vi "handle HTTP Error.vi"(8 "Status String":string, 9 "status code":u16, 11 "error in (no error)":errorcluster) -> (1 "status code dup":u16, 3 "error out":errorcluster)   [LabVIEW 2025, in "http-client.lvclass"]
uses:
  http-client.lvclass
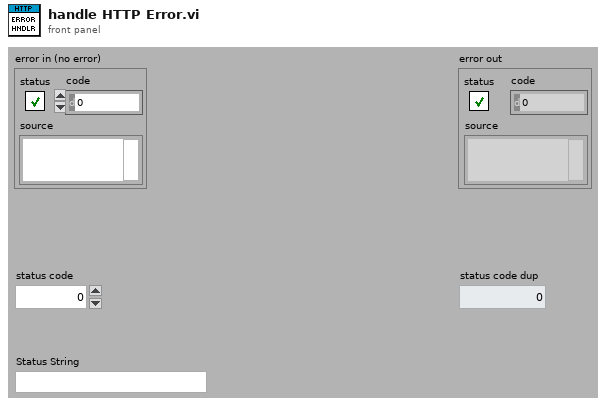
[diagram p1: front panel]
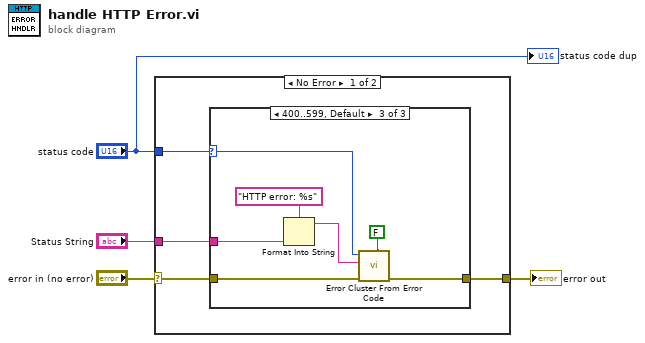
[diagram p0: block diagram]
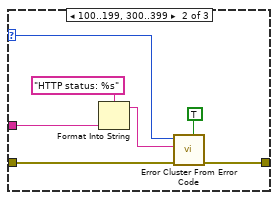
[diagram p3: hidden frame]
diagram:
  n1 = case shown="No Error" "error in (no error)" {
    selector: "error in (no error)" -> [w6 w24]
    tunnel: [w5 w24] -> w3
    tunnel: "status code" -> [w8 _]
    tunnel: "Status String" -> [w7 _]
    frame No Error {
      n2 = case shown="400..599, Default" w8 {
        selector: w8 -> [_ w14 w23]
        tunnel: w7 -> [_ w10 w19]
        tunnel: w6 -> [w9 w15 w18]
        tunnel: [w9 w16 w17] -> w5
        frame 200..299 {
          # "Expected response"
        }
        frame 100..199, 300..399 {
          n3 = Format Into String(format string="HTTP status: %s", w10) -> (resulting string=w11:string)  [unwired: 2 in, 1 out]
          n4 = call <vilib>:"Error Cluster From Error Code.vi"("is warning? (False)"=TRUE, "error in (no error)"=w15, "error message (\"\")"=w11, "error code (0)"=w14) -> ("error out"=w16:errorcluster)  [unwired: 5 in]
        }
        frame 400..599, Default {
          n5 = Format Into String(format string="HTTP error: %s", w19) -> (resulting string=w20:string)  [unwired: 2 in, 1 out]
          n6 = call <vilib>:"Error Cluster From Error Code.vi"("is warning? (False)"=FALSE, "error in (no error)"=w18, "error message (\"\")"=w20, "error code (0)"=w23) -> ("error out"=w17:errorcluster)  [unwired: 5 in]
        }
      }
    }
    frame Error {
    }
  }
  "error out" <- w3
  "status code dup" <- "status code"
